vi "Queue Driver.vi"(0 "Queue Name":string, 5 "State":string, 7 "States[]":string[](array[string]), 11 "Error In":errorcluster, 13 "Queue Operations":T1) -> (4 "Dequeued Element":string, 15 "Error Out":errorcluster)   [LabVIEW 2021, in "Calculator.lvlib"]
doc: "This VI acts as a queue driver , which handles the queue operations such as enqueue ,dequeue , Create, flush and release."
uses:
  Calculator.lvlib
  Controls/Queue Operations.ctl
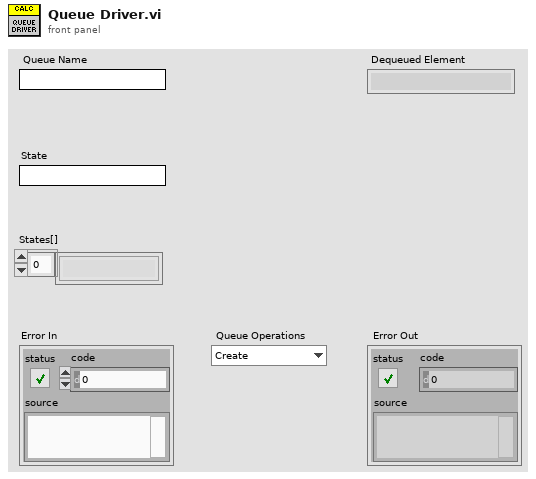
[diagram p1: front panel]
types:
  T1 = typedef "Calculator.lvlib/Queue Operations.ctl" = enum16{"Create", "Enqueue", "EnqueueN", "Enqueue at top", "Dequeue", "Flush", "Release"}
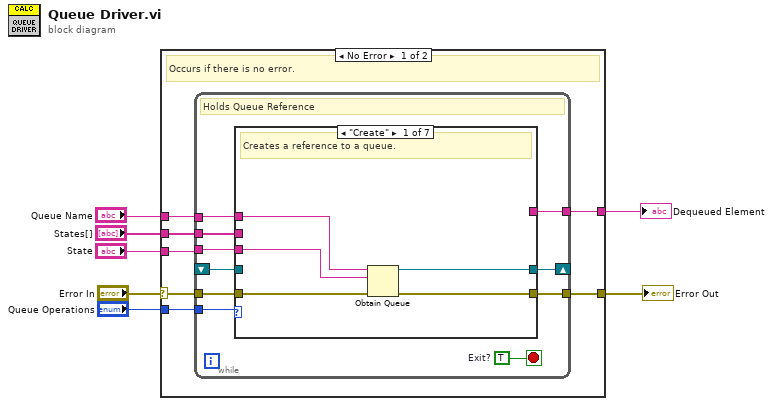
[diagram p0: block diagram]
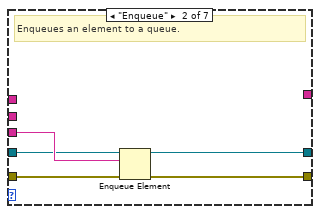
[diagram p2: hidden frame]
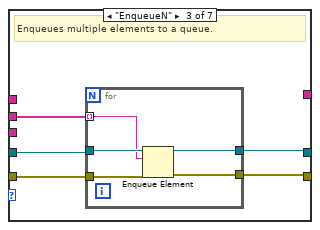
[diagram p3: hidden frame]
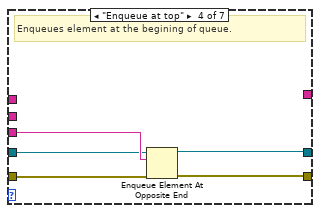
[diagram p4: hidden frame]
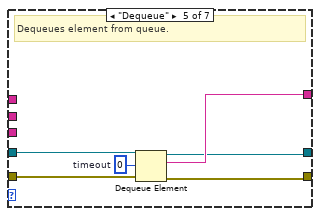
[diagram p5: hidden frame]
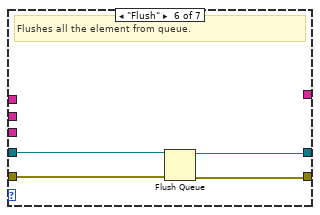
[diagram p6: hidden frame]
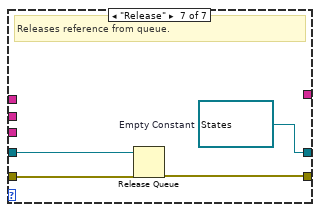
[diagram p7: hidden frame]
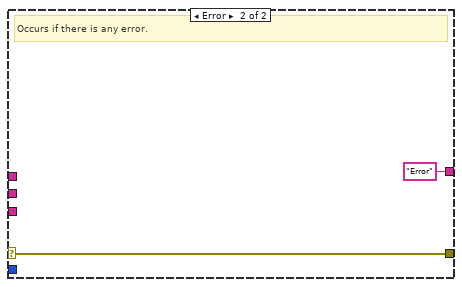
[diagram p8: hidden frame]
diagram:
  n1 = case shown="No Error" "Error In" {
    selector: "Error In" -> [w14 w65]
    tunnel: "Queue Operations" -> [w13 _]
    tunnel: "Queue Name" -> [w12 _]
    tunnel: "State" -> [w11 _]
    tunnel: [w10 "Error" ("States")] -> w3
    tunnel: [w9 w65] -> w2
    tunnel: "States[]" -> [w8 _]
    frame No Error {
      # "Occurs if there is no error."
      n2 = while {
        tunnel: w14 -> [w24]
        tunnel: w13 -> [w23]
        tunnel: w12 -> [w22]
        tunnel: [w21] -> w9
        tunnel: w11 -> [w20]
        shift-right: [w19] -> _
        shift-left: _ -> [w18]
        tunnel: [w17] -> w10
        tunnel: w8 -> [w15]
        stop <- w16 stop-if-true
        w16 = TRUE  # Exit?
        # "Holds Queue Reference"
        n3 = case shown="\"Create\"" w23 {
          tunnel: w22 -> [w29 _ _ _ _ _ _]
          tunnel: w24 -> [w28 w34 w39 w49 w55 w59 w63]
          tunnel: [w25 w30 w38 w45 w51 w56 w62] -> w21
          tunnel: w20 -> [w27 w33 _ w48 _ _ _]
          tunnel: [w26 w32 w36 w47 w52 w57 w60] -> w19
          tunnel: w18 -> [_ w31 w37 w46 w53 w58 w61]
          tunnel: [_ _ _ _ w54 _ _] -> w17
          tunnel: w15 -> [_ _ w35 _ _ _ _]
          frame "Create" {
            # "Creates a reference to a queue."
            n4 = Obtain Queue(name (unnamed)=w29, element data type=w27, error in (no error)=w28) -> (queue out=w26:refnum<queue>, error out=w25:errorcluster)  [unwired: 2 in, 1 out]
          }
          frame "Enqueue" {
            # "Enqueues an element to a queue."
            n5 = Enqueue Element(queue=w31, element=w33, error in (no error)=w34) -> (queue out=w32:refnum<queue>, error out=w30:errorcluster)  [unwired: 1 in, 1 out]
          }
          frame "EnqueueN" {
            # "Enqueues multiple elements to a queue."
            n6 = for {
              tunnel: w39 -> [w44]
              tunnel: [w43] -> w38
              tunnel: w35 -> [w40] mode=indexing
              tunnel: w37 -> [w42]
              tunnel: [w41] -> w36
              n7 = Enqueue Element(queue=w42, element=w40, error in (no error)=w44) -> (queue out=w41:refnum<queue>, error out=w43:errorcluster)  [unwired: 1 in, 1 out]
            }
          }
          frame "Enqueue at top" {
            # "Enqueues element at the begining of queue."
            n8 = Enqueue Element At Opposite End(queue=w46, element=w48, error in (no error)=w49) -> (queue out=w47:refnum<queue>, error out=w45:errorcluster)  [unwired: 1 in, 1 out]
          }
          frame "Dequeue" {
            w50 = 0  # timeout
            # "Dequeues element from queue."
            n9 = Dequeue Element(queue=w53, timeout in ms (-1)=w50, error in (no error)=w55) -> (queue out=w52:refnum<queue>, element=w54:string, error out=w51:errorcluster)  [unwired: 1 out]
          }
          frame "Flush" {
            # "Flushes all the element from queue."
            n10 = Flush Queue(queue=w58, error in (no error)=w59) -> (queue out=w57:refnum<queue>, error out=w56:errorcluster)  [unwired: 1 out]
          }
          frame "Release" {
            w60 = refnum<queue> refnum  # Empty Constant
            # "Releases reference from queue."
            n11 = Release Queue(queue=w61, error in (no error)=w63) -> (error out=w62:errorcluster)  [unwired: 1 in, 2 out]
          }
        }
      }
    }
    frame Error {
      # "Occurs if there is any error."
    }
  }
  "Error Out" <- w2
  "Dequeued Element" <- w3
